vi "AoA Detection 2nd TX Target Signal.vi"() -> ()   [LabVIEW 2015]
doc: "Continuously generates a communication signal that starts immediately. The device is not synchronized to external reference clocks or time bases."
uses:
  <instrlib>/niUSRP/niUSRP Write Tx Data (CDB).vi
  <vilib>/measure/NI_MABase.lvlib
panel:
  out "TX1":bool
  out "TX2":bool
  out "coerced gain":dbl format="%#_6f"
  in  "device names":refnum<k15>="192.168.10.7"
  in  "active antenna":string="TX1"
  in  "tone frequency":dbl=100000.0 format="%#_6p"
  out "Waveform Graph":waveform(dbl)[](graph)
  in  "waveform size":dbl=10000.0
  in  "timeout":dbl=10.0
  out "error out":errorcluster
  in  "stop":bool
  out "coerced carrier frequency":dbl format="%#_6p"
  out "coerced IQ rate":dbl format="%#_6p"
  in  "gain":dbl=30.0 format="%#_6f"
  in  "carrier frequency":dbl=900000000.0 format="%#_6p"
  in  "IQ rate":dbl=1000000.0 format="%#_6p"
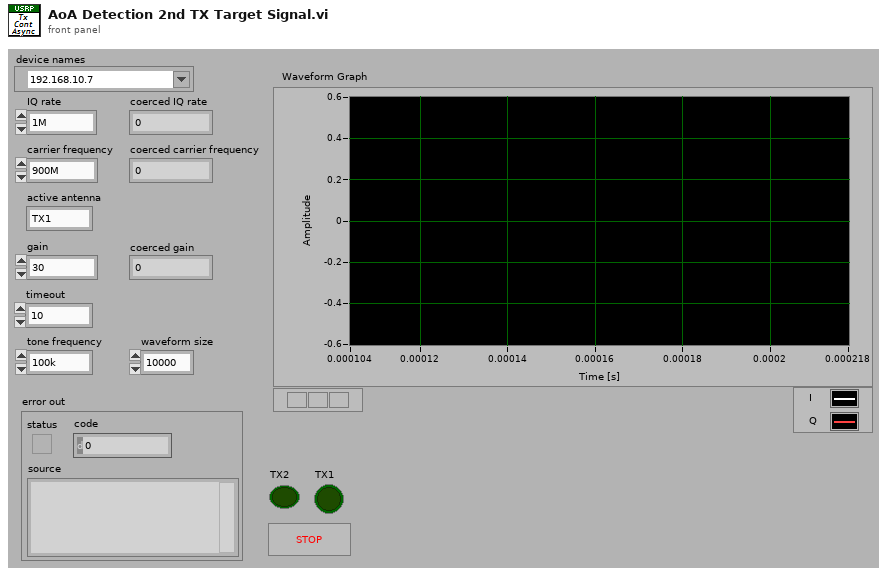
[diagram p1: front panel]
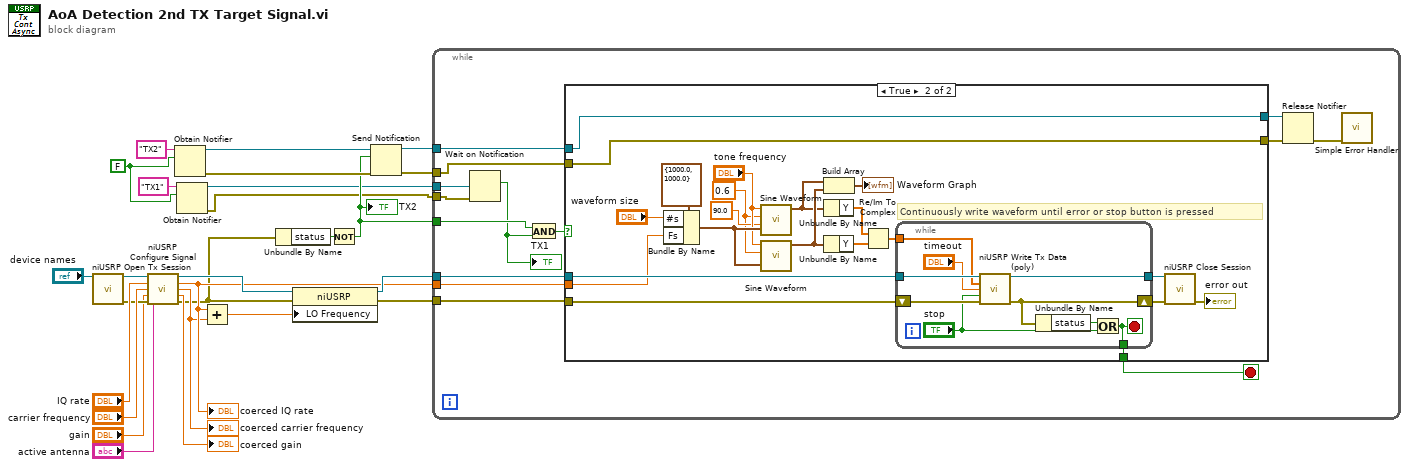
[diagram p0: block diagram]
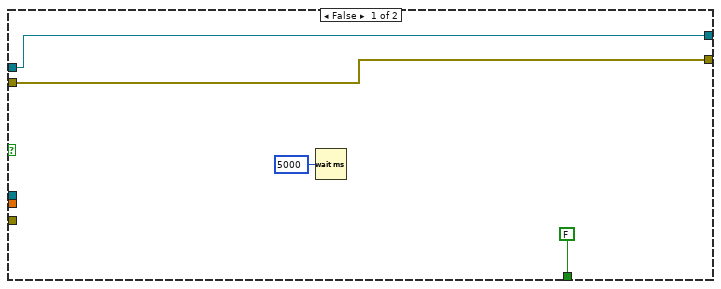
[diagram p2: hidden frame]
diagram:
  w2 = FALSE ("create if not found? (T)")
  n1 = call <instrlib>:"niUSRP Open Tx Session.vi"("device names"="device names") -> ("session handle out"=w26:refnum<k15>, "error out"=w23:errorcluster)  [unwired: 13 in]
  n2 = call <instrlib>:"niUSRP Configure Signal.vi"("session handle"=w26, "IQ rate"="IQ rate", "carrier frequency"="carrier frequency", "gain"="gain", "error in (no error)"=w23, "active antenna"="active antenna") -> ("session handle out"=w17:refnum<k15>, "coerced IQ rate"=w14:dbl, "coerced carrier frequency"=w13:dbl, "coerced gain"=→"coerced gain":dbl, "error out"=w11:errorcluster)  [unwired: 5 in]
  "coerced IQ rate" <- w14
  "coerced carrier frequency" <- w13
  n3 = Obtain Notifier(name (unnamed)="TX2", notification data type=w2) -> (notifier out=w8:refnum<notifier>, error out=w9:errorcluster)  [unwired: 2 in, 1 out]
  n4 = Obtain Notifier(name (unnamed)="TX1", notification data type=w2) -> (notifier out=w4:refnum<notifier>, error out=w3:errorcluster)  [unwired: 2 in, 1 out]
  n5 = Add(x=w14, y=w13) -> (x+y=w15:dbl)
  n6 = Unbundle By Name(w11) -> ("status"=w12:bool)
  n7 = property class="niUSRP"(reference=w17, error in=w11, "LO Frequency"=w15) -> (reference out=w16:refnum<k15>, error out=w18:errorcluster)
  n8 = Not(x=w12) -> (.not. x?=w7:bool)
  "TX2" <- w7
  n9 = Send Notification(notification=w7, notifier=w8, error in (no error)=w9) -> (notifier out=w6:refnum<notifier>, error out=w1:errorcluster)
  n10 = while {
    tunnel: w18 -> [w40]
    tunnel: w16 -> [w39]
    tunnel: w14 -> [w38]
    tunnel: w7 -> [w36]
    tunnel: w6 -> [w30]
    tunnel: w4 -> [w33]
    tunnel: w3 -> [w32]
    tunnel: w1 -> [w28]
    stop <- w37 stop-if-true
    n11 = Wait on Notification(notifier=w33, error in (no error)=w32) -> (notification=w31:bool)  [unwired: 2 in, 3 out]
    "TX1" <- w31
    n12 = And(x=w36, y=w31) -> (x .and. y?=w35:bool)
    n13 = case shown="True" w35 {
      tunnel: w40 -> [_ w64]
      tunnel: w39 -> [_ w50]
      tunnel: w38 -> [_ w48]
      tunnel: [FALSE w47] -> w37
      tunnel: w30 -> [w42 w46]
      tunnel: [w42 w46] -> w29
      tunnel: w28 -> [w41 w45]
      tunnel: [w41 w45] -> w27
      frame False {
        n14 = Wait (ms)(milliseconds to wait=u32 5000) -> ()  [unwired: 1 out]
      }
      frame True {
        w51 = 0.6 ("amplitude")
        # "Continuously write waveform until error or stop button is pressed"
        n15 = Bundle By Name(cluster=cluster{"Fs":dbl, "#s":dbl} {"Fs"=1000.0, "#s"=1000.0} ("sampling info"), "#s"="waveform size", "Fs"=w48) -> (w60:cluster{"Fs":dbl, "#s":dbl})
        n16 = call <vilib>:"Sine Waveform.vi"("sampling info"=w60, "phase"=90.0, "amplitude"=w51, "frequency"="tone frequency") -> ("signal out"=w57:waveform(dbl))  [unwired: 6 in, 1 out]
        n17 = call <vilib>:"Sine Waveform.vi"("sampling info"=w60, "amplitude"=w51, "frequency"="tone frequency") -> ("signal out"=w58:waveform(dbl))  [unwired: 7 in, 1 out]
        n18 = Build Array(w57, w58) -> (→"Waveform Graph":waveform(dbl)[])
        n19 = Unbundle By Name(w57) -> ("Y"=w56:dbl[])
        n20 = Unbundle By Name(w58) -> ("Y"=w55:dbl[])
        n21 = Re/Im To Complex(1:w55, 2:w56) -> (0:w53:cdb[])
        n22 = while {
          tunnel: w50 -> [w74]
          tunnel: [w71] -> w63
          shift-right: [w70] -> w62
          shift-left: w64 -> [w73]
          tunnel: w53 -> [w69]
          tunnel: [w66] -> w47
          stop <- w66 stop-if-true
          n23 = call-poly <instrlib>:"niUSRP Write Tx Data (poly).vi"("session handle"=w74, "data"=w69, "timeout"="timeout", "end of data?"="stop", "error in (no error)"=w73) -> ("session handle out"=w71:refnum<k15>, "error out"=w70:errorcluster)  [unwired: 9 in]
          n24 = Unbundle By Name(w70) -> ("status"=w67:bool)
          n25 = Or(x=w67, y="stop") -> (x .or. y?=w66:bool)
        }
        n26 = call <instrlib>:"niUSRP Close Session.vi"("session handle"=w63, "error in (no error)"=w62) -> ("error out"=→"error out":errorcluster)  [unwired: 13 in]
      }
    }
    n27 = Release Notifier(notifier=w29, error in (no error)=w27) -> (error out=w34:errorcluster)  [unwired: 1 in, 2 out]
    n28 = call <vilib>:"Simple Error Handler.vi"("error in (no error)"=w34) -> ()  [unwired: 4 in, 5 out]
  }
